vi "Cannon Fix.vi"(1 "Cannon Info Modified":T2, 2 "Cannon Info Original":T2) -> (0 "Cannon Info Fixed":T2)   [LabVIEW 2013]
uses:
  <vilib>/Rock Robotics/WPI/Relay/WPI_RelayValue.ctl
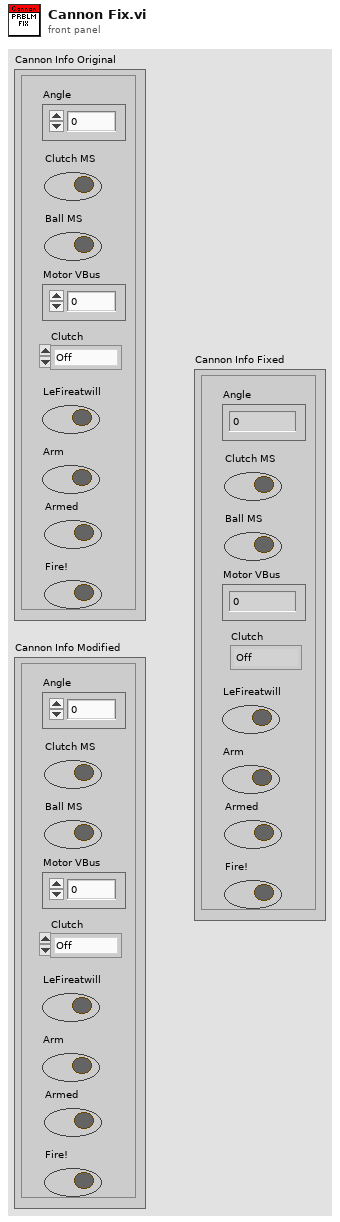
[diagram p1: front panel]
types:
  T1 = typedef "WPI_RelayValue.ctl" = enum16{"Off", "On", "Forward", "Reverse"}
  T2 = cluster{"Angle":dbl, "Clutch MS":bool, "Ball MS":bool, "Motor VBus":dbl, "Clutch ":T1, "LeFireatwill":bool, "Arm":bool, "Armed":bool, "Fire!":bool}
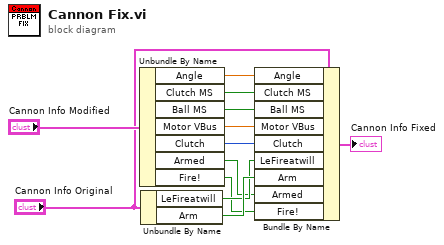
[diagram p0: block diagram]
diagram:
  n1 = Unbundle By Name("Cannon Info Modified") -> ("Angle"=w5:dbl, "Clutch MS"=w4:bool, "Ball MS"=w3:bool, "Motor VBus"=w6:dbl, "Clutch"=w7:T1, "Armed"=w2:bool, "Fire!"=w1:bool)
  n2 = Unbundle By Name("Cannon Info Original") -> ("LeFireatwill"=w8:bool, "Arm"=w9:bool)
  n3 = Bundle By Name(cluster="Cannon Info Original", "Angle"=w5, "Clutch MS"=w4, "Ball MS"=w3, "Motor VBus"=w6, "Clutch"=w7, "LeFireatwill"=w8, "Arm"=w9, "Armed"=w2, "Fire!"=w1) -> (→"Cannon Info Fixed":T2)
